vi "Store Static VI References for Subpanel.vi"(8 "error in (no error)":errorcluster, 11 "Controller Configuration in":refnum<class "MotionSystem Configuration.lvclass">) -> (0 "error out":errorcluster, 3 "Controller Configuration out":refnum<class "MotionSystem Configuration.lvclass">)   [LabVIEW 2016, in "MotionSystem.lvlib" / "MotionSystem Configuration.lvclass"]
uses:
  <userlib>/Common Components/Hardware/Abstract System/MotionSystem/MotionSystem Config/MotionSystem Configuration.lvclass
  C:/Program Files (x86)/National Instruments/LabVIEW 2016/user.lib/Configuration Dialog Actor/Configuration.lvclass
  <userlib>/Common Components/Hardware/Abstract System/MotionSystem/MotionSystem Config/MotionSystem Configuration.lvclass/MotionSystem Configuration.ctl
  <userlib>/Configuration Dialog Actor/Configuration.lvclass/Configuration.ctl
  <userlib>/Configuration Dialog Actor/Accessors/Write Change Display.vi
  <userlib>/Configuration Dialog Actor/Accessors/Write Sub Panel.vi
  <userlib>/Configuration Dialog Actor/Accessors/Write Title.vi
  <userlib>/Common Components/Hardware/Abstract System/MotionSystem/MotionSystem Config/Accessors/Read Array of Motor Configuration Objs.vi
  <userlib>/Configuration Dialog Actor/Accessors/Read Change Display.vi
  <userlib>/Configuration Dialog Actor/Accessors/Read Sub Panel.vi
  <userlib>/Configuration Dialog Actor/Accessors/Read Title.vi
  <userlib>/Common Components/Hardware/Abstract System/MotionSystem/MotionSystem Config/Accessors/Write Array of Motor Configuration Objs.vi
  <userlib>/Common Components/Hardware/Abstract System/MotionSystem/MotionSystem Config/Accessors/Write Array of Motor Category Strings.vi
  <userlib>/Common Components/Hardware/Motor/Motor Config/Motor Configuration.lvclass
  <userlib>/Configuration Dialog Actor/Configuration.lvclass
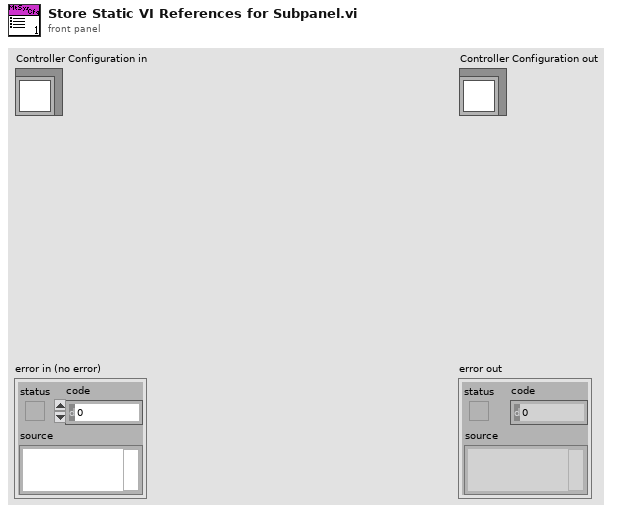
[diagram p1: front panel]
types:
  T1 = typedef "Configuration.lvlib/Configuration.lvclass/Data Retrieved by Lookup Table.ctl" = cluster{"VI Refnum":refnum<vi>, "Help Text":string}
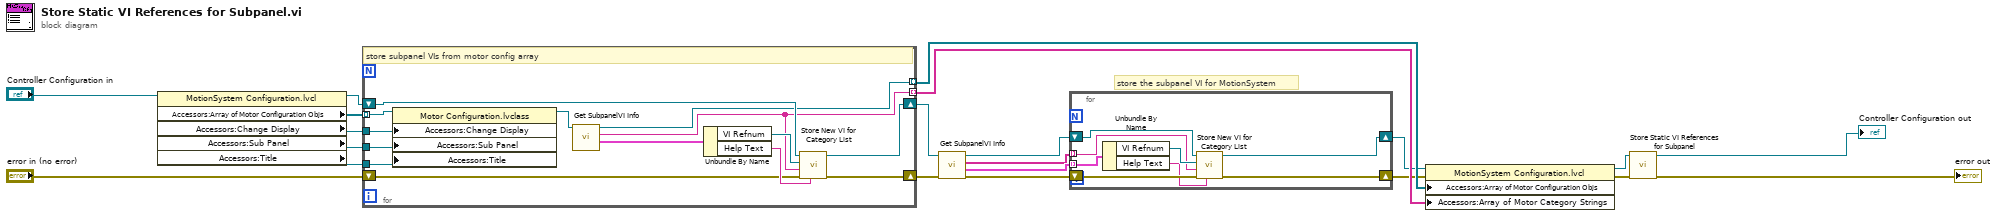
[diagram p0: block diagram]
diagram:
  # "store the subpanel VI for MotionSystem"
  n1 = property class="MotionSystem Configuration.lvcl"(reference="Controller Configuration in") -> (reference out=w18:refnum<class "MotionSystem Configuration.lvclass">, "Accessors:Array of Motor Configuration Objs"=w8:refnum<class "Motor Configuration.lvclass">[], "Accessors:Change Display"=w11:refnum<user-event>, "Accessors:Sub Panel"=w10:refnum<vi>, "Accessors:Title"=w9:refnum<vi>)  [unwired: 1 in, 1 out]
  n2 = for {
    shift-right: [w34] -> w6
    shift-left: w18 -> [w35]
    shift-right: [w29] -> w16
    shift-left: "error in (no error)" -> [w30]
    tunnel: [w27] -> w13 mode=indexing
    tunnel: [w26] -> w12 mode=indexing
    tunnel: w11 -> [w25]
    tunnel: w10 -> [w24]
    tunnel: w9 -> [w23]
    tunnel: w8 -> [w22] mode=indexing
    # "store subpanel VIs from motor config array"
    n3 = property class="Motor Configuration.lvclass"(reference=w22, "Accessors:Change Display"=w25, "Accessors:Sub Panel"=w24, "Accessors:Title"=w23) -> (reference out=w28:refnum<class "Motor Configuration.lvclass">)  [unwired: 1 in, 1 out]
    n4 = call-dynamic "Get SubpanelVI Info.vi"("Motor Configuration in"=w28) -> ("Subpanel VI data"=w33:T1, "Category string"=w26:string, "Motor Configuration out"=w27:refnum<class "Motor Configuration.lvclass">)  [unwired: 7 in, 1 out]
    n5 = Unbundle By Name(w33) -> ("VI Refnum"=w32:refnum<vi>, "Help Text"=w31:string)
    n6 = call <userlib>:"Store New VI for Category List.vi"("Help Text"=w31, "error in (no error)"=w30, "String"=w26, "VI Refnum"=w32, "Configuration in"=w35) -> ("error out"=w29:errorcluster, "Configuration out"=w34:refnum<class "MotionSystem Configuration.lvclass">)  [unwired: 5 in]
  }
  n7 = call-dynamic "Get SubpanelVI Info.vi"("error in (no error)"=w16, "MotionSystem Configuration in"=w6) -> ("error out"=w7:errorcluster, "Array of Subpanel VI data"=w2:T1[], "Array of Category string"=w1:string[], "MotionSystem Configuration out"=w4:refnum<class "MotionSystem Configuration.lvclass">)  [unwired: 6 in]
  n8 = for {
    tunnel: w2 -> [w39] mode=indexing
    tunnel: w1 -> [w36] mode=indexing
    shift-right: [w42] -> w5
    shift-left: w7 -> [w43]
    shift-right: [w40] -> w3
    shift-left: w4 -> [w41]
    n9 = Unbundle By Name(w39) -> ("VI Refnum"=w38:refnum<vi>, "Help Text"=w37:string)
    n10 = call <userlib>:"Store New VI for Category List.vi"("Help Text"=w37, "error in (no error)"=w43, "String"=w36, "VI Refnum"=w38, "Configuration in"=w41) -> ("error out"=w42:errorcluster, "Configuration out"=w40:refnum<class "MotionSystem Configuration.lvclass">)  [unwired: 5 in]
  }
  n11 = property class="MotionSystem Configuration.lvcl"(reference=w3, error in=w5, "Accessors:Array of Motor Configuration Objs"=w13, "Accessors:Array of Motor Category Strings"=w12) -> (reference out=w14:refnum<class "MotionSystem Configuration.lvclass">, error out=w15:errorcluster)
  n12 = call-parent "Store Static VI References for Subpanel.vi"("error in (no error)"=w15, "Configuration in"=w14) -> ("error out"=→"error out":errorcluster, "Configuration out"=→"Controller Configuration out":refnum<class "MotionSystem Configuration.lvclass">)  [unwired: 8 in]
